vi "Update Width.vi"(11 "State in in":T1) -> (3 "State out":T1)   [LabVIEW 2015, in "Read-Write-Signals.xnode"]
uses:
  Read-Write-Signals.xnode
  State.ctl
  Read-Write-Signals Item.ctl
  Read-Write-Signals Sub Item.ctl
  Read-Write-Signals Sub Item Type.ctl
  Read-Write-Signals Selection.ctl
  Read-Write-Signals Display Selection.ctl
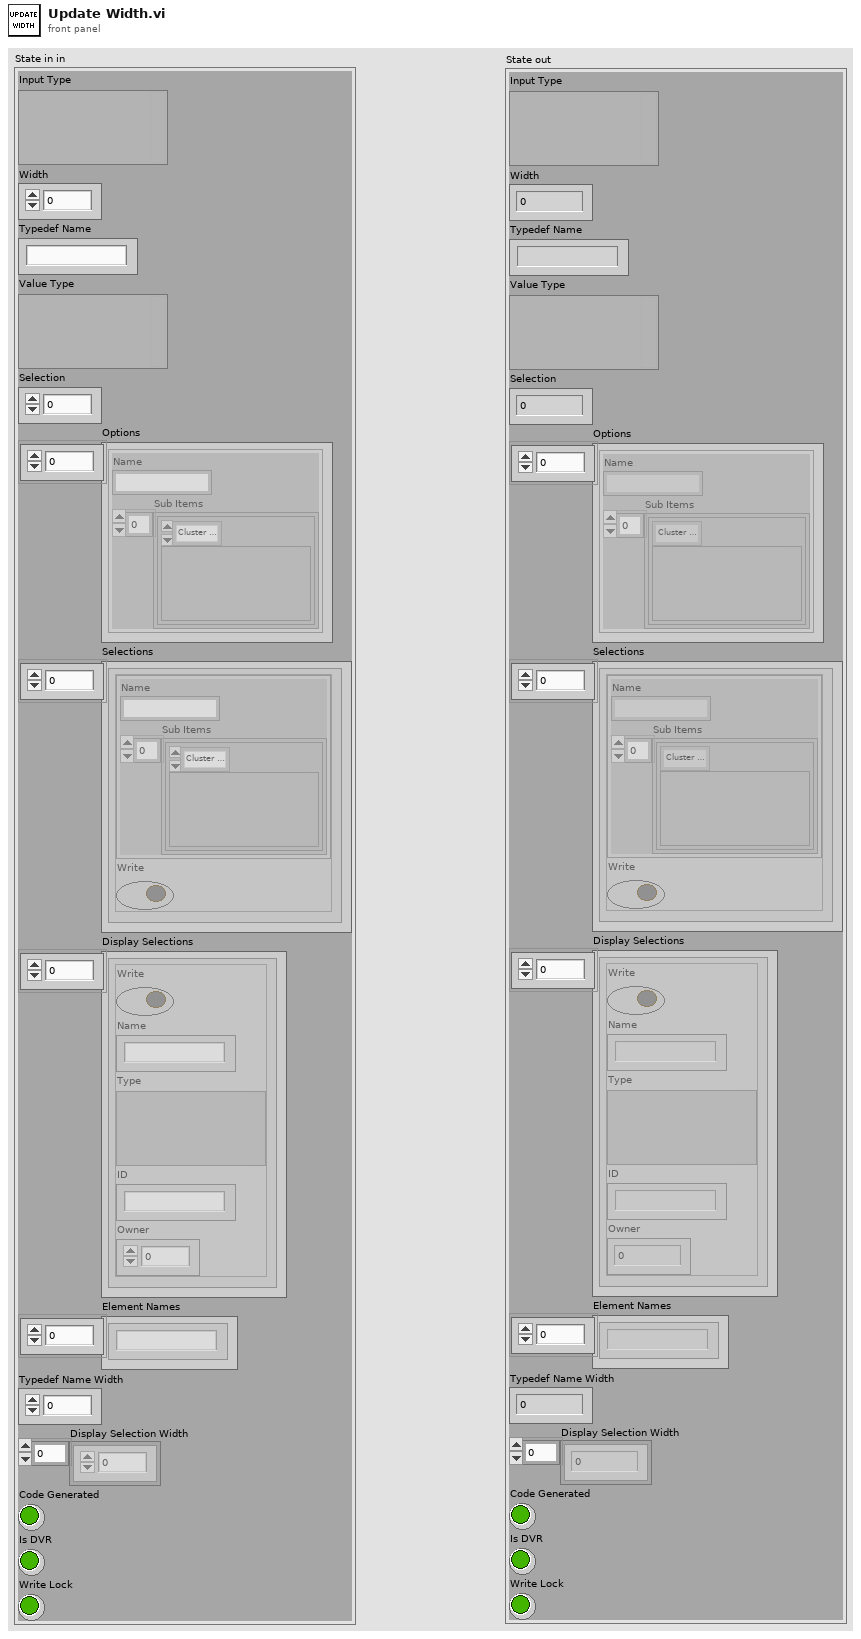
[diagram p1: front panel]
types:
  T1 = typedef "Read-Write-Signals.xnode/State.ctl" = cluster{"Input Type":variant, "Width":i32, "Typedef Name":string, "Value Type":variant, "Selection":i32, "Options":T2[], "Selections":T5[], "Display Selections":T6[], "Element Names":string[], "Typedef Name Width":i32, "Display Selection Width":i32[], "Code Generated":bool, "Is DVR":bool, "Write Lock":bool}
  T2 = typedef "Read-Write-Signals Item.ctl" = cluster{"Name":string, "Sub Items":T3[]}
  T3 = typedef "Read-Write-Signals Sub Item.ctl" = cluster{"Type":T4, "Value":variant}
  T4 = typedef "Read-Write-Signals Sub Item Type.ctl" = enum8{"Cluster Element", "Array Element", "Subarray"}
  T5 = typedef "Read-Write-Signals Selection.ctl" = cluster{"Item":T2, "Write":bool}
  T6 = typedef "Read-Write-Signals Display Selection.ctl" = cluster{"Write":bool, "Name":string, "Type":variant, "ID":string, "Owner":i32}
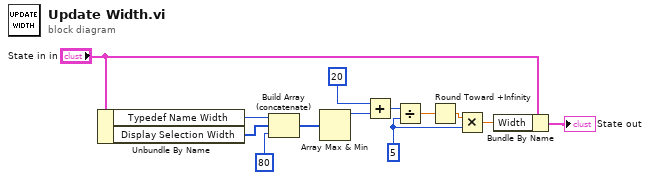
[diagram p0: block diagram]
diagram:
  w2 = 5 ("x")
  n1 = Unbundle By Name("State in in") -> ("Typedef Name Width"=w13:i32, "Display Selection Width"=w12:i32[])
  n2 = Build Array (concatenate)(w13, w12, 80 ("element")) -> (w10:i32[])
  n3 = Array Max & Min(array=w10) -> (max value=w6:i32)  [unwired: 3 out]
  n4 = Add(x=20, y=w6) -> (x+y=w5:i32)
  n5 = Divide(x=w5, y=w2) -> (x/y=w4:dbl)
  n6 = Round Toward +Infinity(x=w4) -> (ceil(x): smallest int >= x=w3:dbl)
  n7 = Multiply(x=w3, y=w2) -> (x*y=w1:dbl)
  n8 = Bundle By Name(cluster="State in in", "Width"=w1) -> (→"State out":T1)
